vi "CAPFM-Init Interval.vi"(0 "Runtime In":T1, 1 "CAPFM Params":T2, 5 "StimChans":T9[](xcontrol), 9 "Interval (ms)":dbl, 11 "error in (no error)":errorcluster) -> (4 "Runtime Out":T1, 15 "error out":errorcluster)   [LabVIEW 2020]
uses:
  epl-vi-lib/Signal Synthesis VIs/Controls/Multichannel (Full)/Multichannel (Full).xctl
  Typedefs/CAPFM-All Params.ctl
  epl-vi-lib/Utility VIs/Type Defs/Left-Right ring.ctl
  Typedefs/CAPFM-Probe Params.ctl
  Typedefs/CAPFM-Masker Params.ctl
  Typedefs/CAPFM-Seq Params.ctl
  Typedefs/CAPFM-Timing Params.ctl
  Typedefs/CAPFM-Response Params.ctl
  Typedefs/CAPFM-Runtime Data.ctl
  epl-vi-lib/Connection VIs/Type Defs/Input sources.ctl
panel:
  out "Waveform Graph":dbl[][](graph)
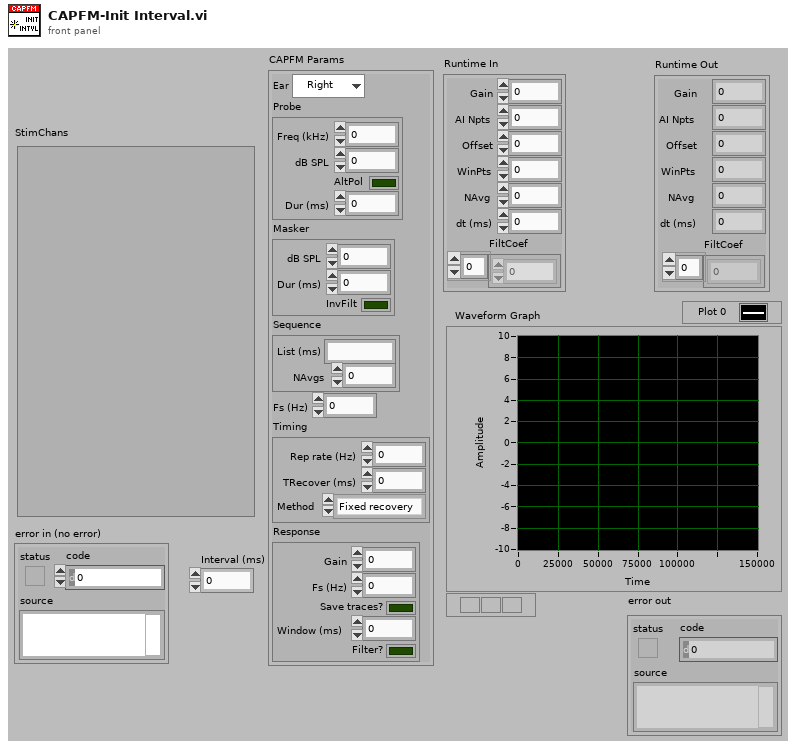
[diagram p1: front panel]
types:
  T1 = typedef "CAPFM-Runtime Data.ctl" = cluster{"Offset":i32, "AI Npts":i32, "Gain":dbl, "WinPts":i32, "NAvg":i32, "dt (ms)":dbl, "FiltCoef":dbl[]}
  T2 = typedef "CAPFM-All Params.ctl" = cluster{"Ear":T3, "Probe":T4, "Masker":T5, "Sequence":T6, "Fs (Hz)":dbl, "Timing":T7, "Response":T8}
  T3 = typedef "Left-Right ring.ctl" = enum16{"Right", "Left"}
  T4 = typedef "CAPFM-Probe Params.ctl" = cluster{"Freq (kHz)":dbl, "dB SPL":dbl, "AltPol":bool, "Dur (ms)":dbl}
  T5 = typedef "CAPFM-Masker Params.ctl" = cluster{"dB SPL":dbl, "Dur (ms)":dbl, "InvFilt":bool}
  T6 = typedef "CAPFM-Seq Params.ctl" = cluster{"List (ms)":string, "NAvgs":i32}
  T7 = typedef "CAPFM-Timing Params.ctl" = cluster{"Rep rate (Hz)":dbl, "TRecover (ms)":dbl, "Method":enum16{"Fixed recovery", "Fixed rep rate"}}
  T8 = typedef "CAPFM-Response Params.ctl" = cluster{"Gain":dbl, "Fs (Hz)":dbl, "Save traces?":bool, "Window (ms)":dbl, "Filter?":bool}
  T9 = typedef "Stimulus Channel (Full).xctl/Full Stimulus Channel Data.ctl" = cluster{"Waveform":T10, "Filter":T27, "Burst":T29, "Level":T30, "Name":string, "Advanced":T32, "SAM":T33}
  T10 = typedef "Waveform XCtl.xctl/Waveform Data.ctl" = cluster{"Type":T11, "Tone":T12, "Pulse Train":T13, "Noise":T16, "File":T17, "FMSweep":T18, "Chirp Train":T19, "Complex Tone":cluster{"Params":T21, "Data":T23}, "Moving Ripple":T24}
  T11 = typedef "Waveform Enum.ctl" = enum16{"OFF", "Tone", "Noise", "Pulse Train", "File", "FM Sweep", "Chirp Train", "Complex Tone", "FM Tone", "Moving Ripple"}
  T12 = typedef "Tone Params.ctl" = cluster{"Frequency (kHz)":dbl, "Last Freq":dbl, "Last Phase":dbl}
  T13 = typedef "Pulse Train Params.ctl" = cluster{"Pulse width (us)":dbl, "Pulse rate (Hz)":dbl, "Gap (ms)":dbl, "Polarity":T14, "PT State":T15, "Asynch":bool}
  T14 = typedef "Pulse Polarity.ctl" = enum16{"POS", "NEG", "POS-NEG", "NEG-POS"}
  T15 = typedef "PT-Continuous State.ctl" = cluster{"Template":dbl[], "Nperiod":i32, "Index":i32, "Pulse Rate (Hz)":dbl, "Phase (cycles)":dbl, "Noff":i32}
  T16 = typedef "Noise Params.ctl" = cluster{"InvFilt":bool, "Noise":dbl[], "CurPt":i32, "Aweight":bool, "Seed":i32, "afile":path}
  T17 = typedef "StimFile-Params.ctl" = cluster{"Filename":path, "Signal":dbl[], "Channel":i32, "stream":bool, "offset":i32, "nreps":i32, "loops":i32, "Randomize":bool, "order":i32[], "Seed":i32, "Tokens":i32}
  T18 = typedef "FM Sweep Params.ctl" = cluster{"Rate (oct/s)":dbl, "Fmin (Hz)":dbl, "Fmax (Hz)":dbl, "Ramp (ms)":dbl, "Linear":bool}
  T19 = typedef "Chirp Train.ctl" = cluster{"Params":T20, "Data":cluster{"WF":dbl[]}}
  T20 = typedef "Chirp Train Params.ctl" = cluster{"Fmin (kHz)":dbl, "Fmax (kHz)":dbl, "Compensate":bool, "Duration (ms)":dbl}
  T21 = typedef "CT-Params.ctl" = cluster{"F0 (Hz)":dbl, "Band":cluster{"Flow (Hz)":dbl, "Fhigh (Hz)":dbl}, "Phase":T22, "Min F0 (Hz)":dbl, "Max F0 (Hz)":dbl, "ContinRandPhase":bool, "Max peak factor":dbl, "Max mod depth":dbl, "MinHarmNum":i32, "MaxHarmNum":i32, "Level Mode":enum16{"per component", "overall rms"}, "% jitter":dbl}
  T22 = typedef "CT-Phase Enum.ctl" = enum16{"Cosine", "Random", "Alternating"}
  T23 = typedef "CT-Runtime Data.ctl" = cluster{"Ncomp":i32, "MinHarm":i32, "Phase":dbl[], "Amplitude":dbl[], "Npts/frame":i32, "Last F0":dbl, "Fmin":dbl, "Fmax":dbl, "Lslope":dbl, "randphase":bool, "overall rms":bool, "fmult":dbl[], "jittered":bool}
  T24 = typedef "Moving Ripple.ctl" = cluster{"Params":T25, "Data":T26}
  T25 = typedef "Moving Ripple.Params.ctl" = cluster{"Fmin":dbl, "Fmax":dbl, "Density":dbl, "Velocity":dbl, "Depth":dbl, "Phase":dbl, "Comp/oct":i32}
  T26 = typedef "Moving Ripple.Data.ctl" = cluster{"Freq":dbl[], "A":dbl[], "phase":dbl[], "Phase":dbl}
  T27 = typedef "Advanced Filter XCtl.xctl/Filter Data.ctl" = cluster{"Type":enum16{"Lowpass", "Highpass", "Bandpass", "Bandstop", "OFF"}, "CF (kHz)":dbl, "BW (kHz)":dbl, "Cascade":bool, "Quadrature":bool, "Scale Factor":dbl, "Stages":cluster{"IIR Filter":cluster{"filter structure":enum32{"IIR 2nd Order", "IIR 4th Order"}, "Reverse Coefficients":dbl[], "Forward Coefficients":dbl[]}, "State":dbl[]}[], "Class":enum16{"Elliptic", "Butterworth"}, "Order":i32, "BWUnits":T28}
  T28 = typedef "Filter-Bandwidth Units.ctl" = enum16{"Linear", "Octaves", "Min-Max"}
  T29 = typedef "Burst Control.xctl/Burst Data.ctl" = cluster{"Active":bool, "Delay (ms)":dbl, "Duration (ms)":dbl, "Ramp (ms)":dbl, "Rate (Hz)":dbl, "Trepeat (ms)":dbl, "Repeat":bool}
  T30 = typedef "Level XCtl.xctl/Level Data.ctl" = cluster{"Level":dbl, "Units":T31, "Max":dbl, "Multiplier":dbl, "Cal File":path, "Cal":cluster{"Freq (Hz)":dbl[], "Mag (dB SPL)":dbl[], "Phase (deg)":dbl[]}}
  T31 = typedef "Level Units.ctl" = enum16{"dB atten", "dB SPL", "dB re 1 Vrms", "dB V/Hz½", "mW", "dB HL", "Volts", "dB mW"}
  T32 = typedef "Advanced Stimulus Options.xctl/Advanced Stimulus Options.ctl" = cluster{"Rep Mask":string, "AltPol":bool, "Var":string, "Expr":string, "Persist":bool}
  T33 = typedef "SAM Params.ctl" = cluster{"Active":bool, "Frequency (Hz)":dbl, "Depth":dbl, "Init Phase (cycles)":dbl, "phase (degrees)":dbl, "Asynch":bool}
  T34 = typedef "Input sources.ctl" = u16
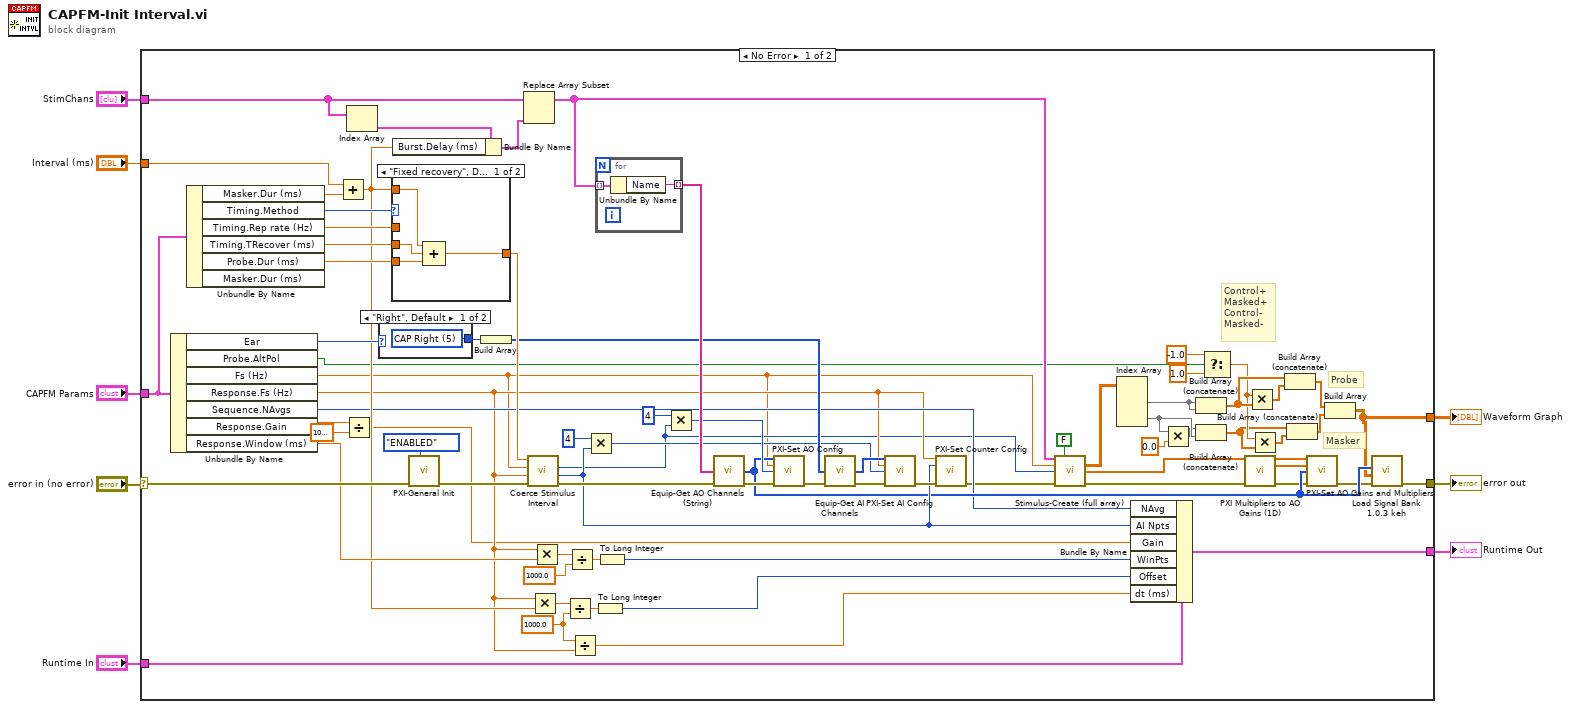
[diagram p0: block diagram]
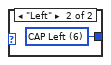
[diagram p2: hidden frame]
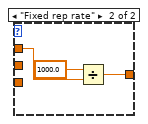
[diagram p3: hidden frame]
diagram:
  n1 = case shown="No Error" "error in (no error)" {
    selector: "error in (no error)" -> [w72 w96]
    tunnel: [w30 w96] -> w7
    tunnel: "CAPFM Params" -> [w77 _]
    tunnel: "Interval (ms)" -> [w84 _]
    tunnel: "StimChans" -> [w83 _]
    tunnel: [w47 _] -> w3
    tunnel: [w17 _] -> w2
    tunnel: "Runtime In" -> [w11 _]
    frame No Error {
      w28 = 1000.0 ("y")
      # "Masker"
      # "Probe"
      # "Control+\nMasked+\nControl-\nMasked-"
      n2 = Unbundle By Name(w77) -> ("Ear"=w64:T3, "Probe.AltPol"=w40:bool, "Fs (Hz)"=w24:dbl, "Response.Fs (Hz)"=w27:dbl, "Sequence.NAvgs"=w29:i32, "Response.Gain"=w57:dbl, "Response.Window (ms)"=w56:dbl)
      n3 = Unbundle By Name(w77) -> ("Masker.Dur (ms)"=w73:dbl, "Timing.Method"=w81:enum16{"Fixed recovery", "Fixed rep rate"}, "Timing.Rep rate (Hz)"=w80:dbl, "Timing.TRecover (ms)"=w78:dbl, "Probe.Dur (ms)"=w79:dbl)  [unwired: 1 out]
      n4 = Add(x=w84, y=w73) -> (x+y=w49:dbl)
      n5 = Divide(x=w57, y=1000000.0) -> (x/y=w16:dbl)
      n6 = Index Array(array=w83) -> (element=w9:T9)  [unwired: 1 in]
      n7 = case shown="\"Right\", Default" w64 {
        tunnel: [w85 w86] -> w63
        frame "Right", Default {
          w85 = T34 5 items=["--unused--", "Probe Mic Right", "Probe Mic Left", "Cal Mic", "ABR", "CAP Right", "CAP Left", "Startle piezo", "Temperature", "Heart rate", "Accelerometer", "Startle piezo 2"] ("Ring")
        }
        frame "Left" {
          w86 = T34 6 items=["--unused--", "Probe Mic Right", "Probe Mic Left", "Cal Mic", "ABR", "CAP Right", "CAP Left", "Startle piezo", "Temperature", "Heart rate", "Accelerometer", "Startle piezo 2"] ("Ring")
        }
      }
      n8 = case shown="\"Fixed recovery\", Default" w81 {
        tunnel: w80 -> [_ w95]
        tunnel: w79 -> [w90 _]
        tunnel: w49 -> [w92 _]
        tunnel: w78 -> [w91 _]
        tunnel: [w89 w94] -> w69
        frame "Fixed recovery", Default {
          n9 = Compound Arithmetic op=ADD(w92, w91, w90) -> (w89:dbl)
        }
        frame "Fixed rep rate" {
          n10 = Divide(x=1000.0, y=w95) -> (x/y=w94:dbl)
        }
      }
      n11 = Bundle By Name(cluster=w9, "Burst.Delay (ms)"=w49) -> (w82:T9)
      n12 = call "PXI-General Init.vi"("Double Buffer Mode"=enum32{"OFF", "ENABLED", "FORCED"}."ENABLED", "error in (no error)"=w72) -> ("error out"=w71:errorcluster)  [unwired: 9 in]
      n13 = Build Array(w63) -> (w62:T34[])
      n14 = Replace Array Subset(array=w83, new element=w82) -> (w45:T9[])  [unwired: 1 in]
      n15 = call "Coerce Stimulus Interval.vi"("error in (no error)"=w71, "AI sampling rate (Hz)"=w27, "AO sampling rate (Hz)"=w24, "Stimulus interval (ms)"=w69) -> ("error out"=w70:errorcluster, "AI npts"=w46:i32, "AO npts"=w25:i32)  [unwired: 4 in, 1 out]
      n16 = Multiply(x=w27, y=w49) -> (x*y=w51:dbl)
      n17 = Multiply(x=w27, y=w56) -> (x*y=w55:dbl)
      n18 = Divide(x=w51, y=w28) -> (x/y=w50:dbl)
      n19 = Divide(x=w55, y=1000.0) -> (x/y=w53:dbl)
      n20 = Divide(x=w28, y=w27) -> (x/y=w26:dbl)
      n21 = Multiply(x=4, y=w46) -> (x*y=w59:i32)
      n22 = To Long Integer(number=w50) -> (32bit integer=w48:i32)
      n23 = for {
        tunnel: w45 -> [w88] mode=indexing
        tunnel: [w87] -> w74 mode=indexing
        n24 = Unbundle By Name(w88) -> ("Name"=w87:string)
      }
      n25 = To Long Integer(number=w53) -> (32bit integer=w52:i32)
      n26 = Multiply(x=4, y=w25) -> (x*y=w68:i32)
      n27 = call "Equip-Get AO Channels (String).vi"("Channel Names"=w74, "error in (no error)"=w70) -> ("AO Channels"=w36:i32[], "error out"=w75:errorcluster)  [unwired: 12 in]
      n28 = call "PXI-Set AO Config.vi"("AO Channels"=w36, "Sampling Rate (Hz)"=w24, "Buffer Size"=w68, "error in (no error)"=w75) -> ("error out"=w65:errorcluster)  [unwired: 11 in]
      n29 = call "Equip-Get AI Channels.vi"("Inputs"=w62, "error in (no error)"=w65) -> ("AI Channels"=w61:i32[], "error out"=w60:errorcluster)  [unwired: 12 in]
      n30 = call "PXI-Set AI Config.vi"("AI Channels"=w61, "Sampling Rate (Hz)"=w27, "Buffer Size"=w59, "error in (no error)"=w60) -> ("error out"=w58:errorcluster)  [unwired: 11 in]
      n31 = call "PXI-Set Counter Config.vi"("AI Sampling Rate (Hz)"=w27, "Num AI Pts"=w46, "error in (no error)"=w58) -> ("error out"=w12:errorcluster)  [unwired: 12 in]
      n32 = call "Stimulus-Create (full array).vi"("StimChan"=w45, "Apply multipliers? (F)"=FALSE, "Sampling Rate (Hz)"=w24, "Npts"=w25, "error in (no error)"=w12) -> ("Waveform"=w43:dbl[][], "Multipliers"=w14:dbl[], "error out"=w34:errorcluster)  [unwired: 7 in, 1 out]
      n33 = Index Array(array=w43) -> (element #1=w10:dbl[], element #2=w23:dbl[])  [unwired: 4 in]
      n34 = Bundle By Name(cluster=w11, "NAvg"=w29, "AI Npts"=w46, "Gain"=w16, "WinPts"=w52, "Offset"=w48, "dt (ms)"=w26) -> (w47:T1)
      n35 = Multiply(x=w23, y=0.0) -> (x*y=w13:dbl[])
      n36 = Build Array (concatenate)(w10, w10) -> (w41:dbl[])
      n37 = Build Array (concatenate)(w13, w23) -> (w21:dbl[])
      n38 = Select(t=-1.0, s=w40, f=1.0) -> (s? t:f=w22:dbl)
      n39 = call "PXI Multipliers to AO Gains (1D).vi"("Multipliers in"=w14, "error in (no error)"=w34) -> ("Multipliers out"=w33:dbl[], "Gains"=w32:dbl[], "error out"=w31:errorcluster)  [unwired: 11 in]
      n40 = Multiply(x=w22, y=w41) -> (x*y=w37:dbl[])
      n41 = Multiply(x=w22, y=w21) -> (x*y=w20:dbl[])
      n42 = Build Array (concatenate)(w41, w37) -> (w19:dbl[])
      n43 = Build Array (concatenate)(w21, w20) -> (w18:dbl[])
      n44 = call "PXI-Set AO Gains and Multipliers.vi"("Multipliers"=w33, "Gains"=w32, "AO Channels"=w36, "error in (no error)"=w31) -> ("error out"=w35:errorcluster)  [unwired: 11 in]
      n45 = Build Array(w19, w18) -> (w17:dbl[][])
      n46 = call "Load Signal Bank 1.0.3 keh.vi"("error in (no error)"=w35, "Input array"=w17, "Active AO Array"=w36) -> ("error out"=w30:errorcluster)  [unwired: 6 in, 2 out]
    }
    frame Error {
    }
  }
  "error out" <- w7
  "Runtime Out" <- w3
  "Waveform Graph" <- w2
